vi "fpga_Check Sequence Status.vi"(9 "shot count":u8, 10 "shot trip? (F)":bool, 11 "reset to ready state? (F)":bool) -> (3 "sequence timer active?":bool)   [LabVIEW 2012, in "NI_EP_Protection_FPGA.lvlib"]
uses:
  <vilib>/addons/Electrical Power/Protection/NI_EP_Protection_FPGA.lvlib
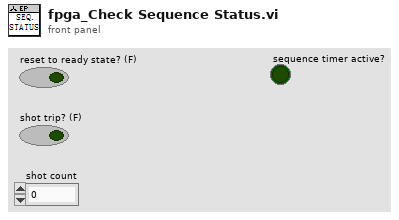
[diagram p1: front panel]
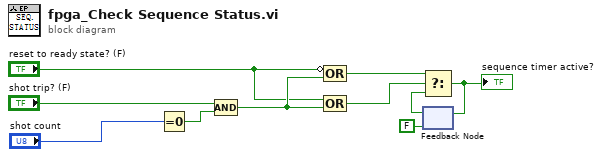
[diagram p0: block diagram]
diagram:
  n1 = Equal To 0?(x="shot count") -> (x = 0?=w6:bool)
  n2 = Compound Arithmetic op=AND("shot trip? (F)", w6) -> (w8:bool)
  n3 = Compound Arithmetic op=OR(invert "reset to ready state? (F)", w8) -> (w3:bool)
  n4 = Compound Arithmetic op=OR("reset to ready state? (F)", w8) -> (w4:bool)
  n5 = feedback #1(FALSE) -> (w1:bool)
  n6 = Select(t=w3, s=w4, f=w1) -> (s? t:f=w2:bool)
  "sequence timer active?" <- w2
  n7 = feedback-in #1(w2) -> ()
